vi "Control Events.vi"(8 "error in (no error)":errorcluster, 11 "DblPopupControl in":refnum<class "DblPopupControl.lvclass">) -> (0 "error out":errorcluster, 2 "Control Events":refnum<class "Control Event Registrations.lvclass">, 3 "DblPopupControl out":refnum<class "DblPopupControl.lvclass">)   [LabVIEW 2020, in "VolatusGUIElements.lvlib" / "DblPopupControl.lvclass"]
uses:
  DblPopupControl.lvclass
  VolatusGUI/Control Event Registrations/Control Event Registrations.lvclass
  DblPopupControl.lvclass/DblPopupControl.ctl
  C:/dev/lv20CE/relink/lv-volatus/VolatusGUI/Control/Control.lvclass
  C:/dev/lv20CE/relink/lv-volatus/VolatusGUI/GUI Element/GUI Element.lvclass
  C:/dev/lv20CE/relink/lv-volatus/VolatusGUIElements/DblPopupControl/DblPopupControl.lvclass
  C:/dev/lv20CE/relink/lv-volatus/VolatusGUI/OnMouseDown/OnMouseDown.lvclass
  VolatusGUI/GUI Element/GUI Element.lvclass
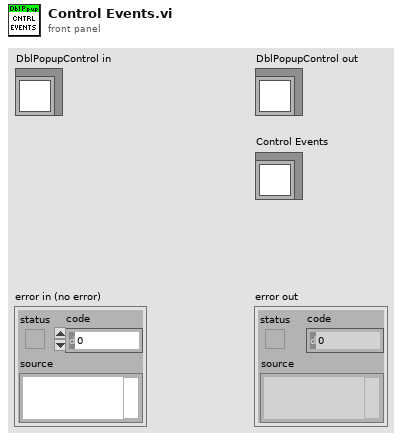
[diagram p1: front panel]
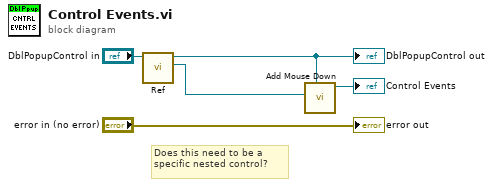
[diagram p0: block diagram]
diagram:
  # "Does this need to be a specific nested control?"
  n1 = call "Ref.vi"("GUI Element in"="DblPopupControl in") -> ("Ref"=w1:refnum<vi>, "GUI Element out"=w2:refnum<class "DblPopupControl.lvclass">)  [unwired: 9 in]
  "DblPopupControl out" <- w2
  n2 = call "Add Mouse Down.vi"("Control"=w2, "CtlRef"=w1) -> ("Control Event Registrations out"=→"Control Events":refnum<class "Control Event Registrations.lvclass">)  [unwired: 8 in, 1 out]
  "error out" <- "error in (no error)"
